vi "Configure VIs.Progress Window.New.vi"(8 "error in (no error)":errorcluster, 11 "VI path":path) -> (0 "error out":errorcluster, 2 "DVRs":T1, 3 "VI refnum":refnum<vi>)   [LabVIEW 2016, in "Memory Manager.lvlib"]
uses:
  Memory Manager.lvlib
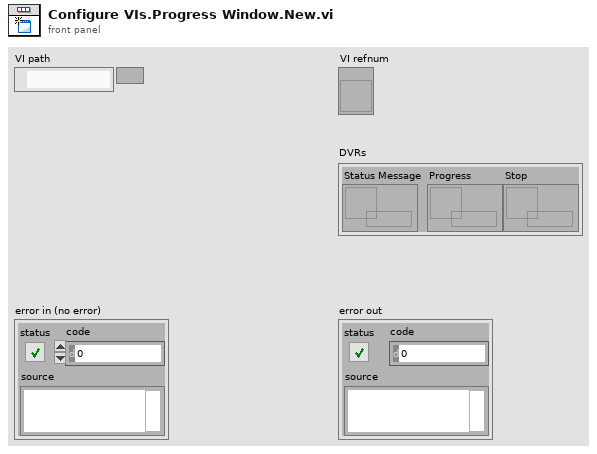
[diagram p1: front panel]
types:
  T1 = cluster{"Status Message":refnum<data-value>, "Progress":refnum<data-value>, "Stop":refnum<data-value>}
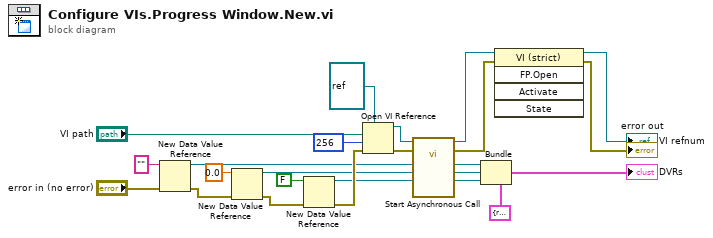
[diagram p0: block diagram]
diagram:
  n1 = New Data Value Reference(data value="", error in="error in (no error)") -> (data value reference=w7:refnum<data-value>, error out=w19:errorcluster)
  n2 = New Data Value Reference(data value=0.0, error in=w19) -> (data value reference=w6:refnum<data-value>, error out=w20:errorcluster)
  n3 = New Data Value Reference(data value=FALSE, error in=w20) -> (data value reference=w8:refnum<data-value>, error out=w11:errorcluster)
  n4 = Open VI Reference(type specifier VI Refnum (for type only)=refnum<vi> refnum, vi path="VI path", options=256, error in (no error)=w11) -> (vi reference=w14:refnum<vi>, error out=w15:errorcluster)  [unwired: 2 in]
  n5 = call-by-ref "Start Asynchronous Call"(reference=w14, error in=w15, "Stop"=w8, "Progress"=w6, "Status String"=w7) -> (reference out=w4:refnum<vi>, error out=w2:errorcluster)  [unwired: 9 in]
  n6 = Bundle(cluster=T1 {"Status Message"=refnum, "Progress"=refnum, "Stop"=refnum} ("DVRs"), "Status Message"=w7, "Progress"=w6, "Stop"=w8) -> (→"DVRs":T1)
  n7 = invoke class="VI (strict)" method="FP.Open"(reference=w4, error in=w2) -> (reference out=→"VI refnum":refnum<vi>, error out=→"error out":errorcluster)  [unwired: 3 in, 3 out]
